vi "DAQmx Timing (Pipelined Sample Clock).vi"(0 "task/channels in":refnum<k21>, 1 "sample mode":i32(ring)=10178 items=["Finite Samples"=10178, "Continuous Samples"=10123, "Hardware Timed Single Point"=12522], 2 "samples per channel":i32=1000, 5 "rate":dbl=1000.0 format="%0.2f", 7 "source":tag, 9 "active edge":i32(ring)=10280 items=["Rising"=10280, "Falling"=10171], 11 "error in":errorcluster) -> (4 "task out":refnum<k21>, 15 "error out":errorcluster)   [LabVIEW 2011]
doc: "Sets the source of the Sample Clock, the rate of the Sample Clock, and the number of samples to acquire or generate. The device acquires or generates samples on each Sample Clock edge, but it does not respond to certain triggers until a few Sample Clock edges later. Pipelining allows higher data transfer rates at the cost of increased trigger response latency. Refer to the device documentation for information about which triggers pipelining affects.\n\nThis timing type allows handshaking using the Pause trigger and either the Ready for Transfer event or the Data Active event. Refer to the device documentation for more information.\n\nThis timing type is supported only by the NI 6536 and NI 6537."
uses:
  C:/Program Files/National Instruments/LabVIEW 2011/resource/objmgr/daqmx.rc
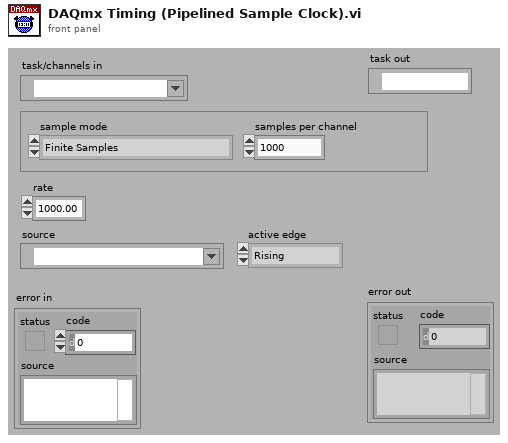
[diagram p1: front panel]
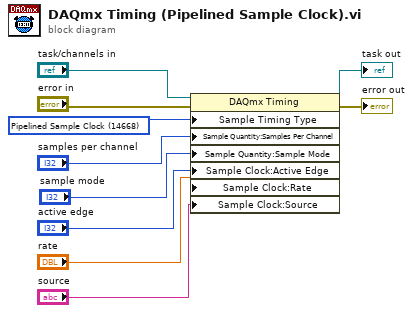
[diagram p0: block diagram]
diagram:
  w1 = 14668 items=["Sample Clock"=10388, "Burst Handshake"=12548, "Handshake"=10389, "Implicit"=10451, "On Demand"=10390, "Change Detection"=12504, "Pipelined Sample Clock"=14668] ("SampTimingType")
  n1 = property class="DAQmx Timing"(reference="task/channels in", error in="error in", "Sample Timing Type"=w1, "Sample Quantity:Samples Per Channel"="samples per channel", "Sample Quantity:Sample Mode"="sample mode", "Sample Clock:Active Edge"="active edge", "Sample Clock:Rate"="rate", "Sample Clock:Source"="source") -> (reference out=→"task out":refnum<k21>, error out=→"error out":errorcluster)
